vi "Updata.vi"(8 "error in (no error)":errorcluster, 11 "DisplayUI in":refnum<class "DisplayUI.lvclass">) -> (0 "error out":errorcluster, 3 "DisplayUI out":refnum<class "DisplayUI.lvclass">)   [LabVIEW 2013, in "DisplayUI.lvclass"]
uses:
  DisplayUI.lvclass
  DisplayUI.lvclass/DisplayUI.ctl
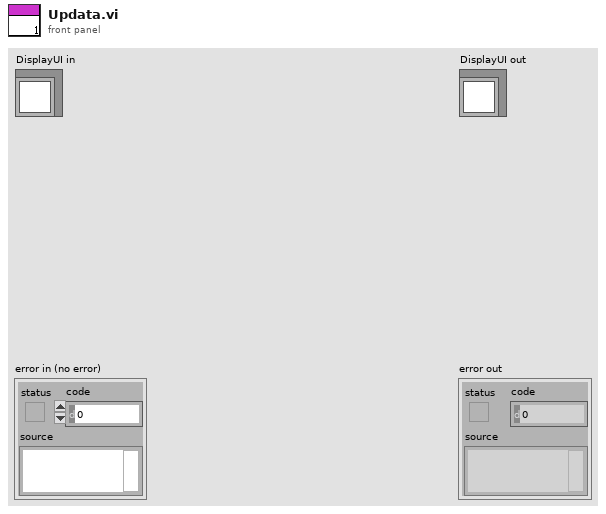
[diagram p1: front panel]
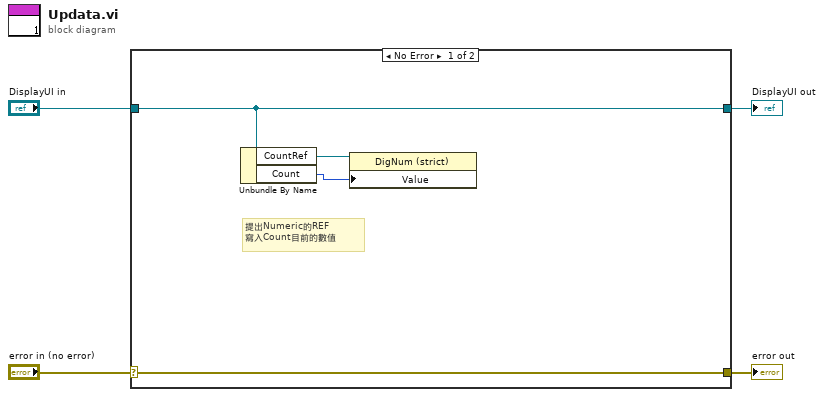
[diagram p0: block diagram]
diagram:
  n1 = case shown="No Error" "error in (no error)" {
    selector: "error in (no error)" -> [w8 w10]
    tunnel: [w8 w10] -> w3
    tunnel: [w7 w9] -> w1
    tunnel: "DisplayUI in" -> [w7 w9]
    frame No Error {
      # "提出Numeric的REF\n寫入Count目前的數值"
      n2 = Unbundle By Name(w7) -> ("CountRef"=w6:refnum<vi>, "Count"=w5:i32)
      n3 = property class="DigNum (strict)"(reference=w6, "Value"=w5) -> ()  [unwired: 1 in, 2 out]
    }
    frame Error {
    }
  }
  "error out" <- w3
  "DisplayUI out" <- w1
